vi "Host Image Acquisition Loop.vi"(8 "error in":errorcluster, 11 "Image Reference":refnum<vi>) -> (0 "error out":errorcluster)   [LabVIEW 2013]
doc: "Loop handles the matlab tcp communications.\nInitialize - Queues up the intialize states\nWait For Connection - Calls the TCP module and waits for a connection to be established\nRead Data - Calls the TCP module and reads the data at the port and then parses the command\nCheck Messages - Checks message queue for external messages sent from other threads\nClose Connection - Closes the TCP connection\nExit"
uses:
  Common/State Machines/State Machine Lib.lvlib
  Message Passing/Main MsgQ.lvlib
  Host Image Acquisition Module Enum.ctl
  Message Passing/MsgQ Loops enum.ctl
panel:
  out "FPGA Image":T1(plugin-control)
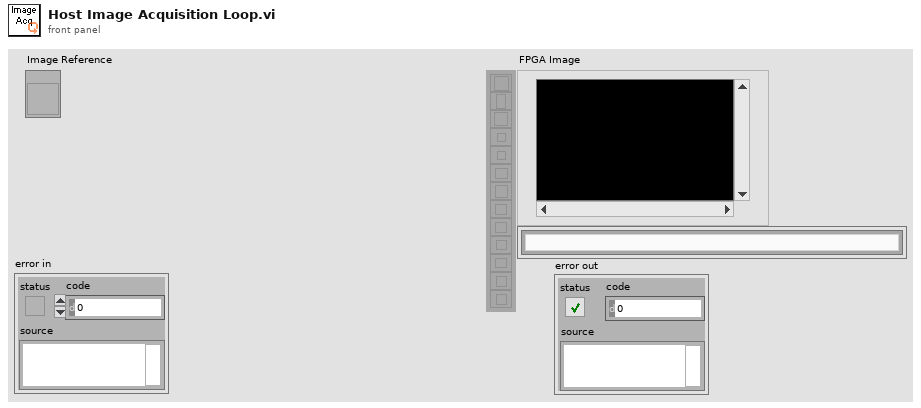
[diagram p1: front panel]
types:
  T1 = typedef "IMAQ Image.ctl" = refnum<image>
  T2 = typedef "State Machine Lib.lvlib/STATE cluster.ctl" = cluster{"State":string, "Parameters":variant}
  T3 = typedef "Host Image Acquisition Module Enum.ctl" = enum16{"Open FPGA", "Initialize DMA FIFO", "Start Acquisition", "Aquire Image", "Close FPGA"}
  T4 = typedef "Main MsgQ.lvlib/MsgQ Loops enum.ctl" = enum16{"User Interface", "Image Acq"}
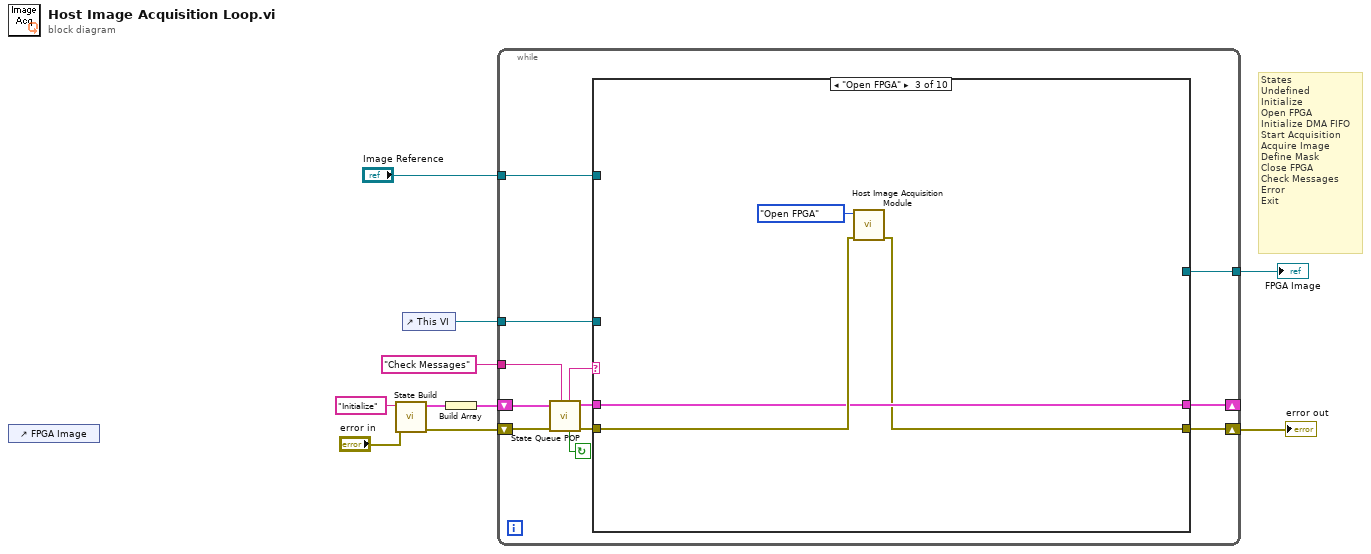
[diagram p0: block diagram]
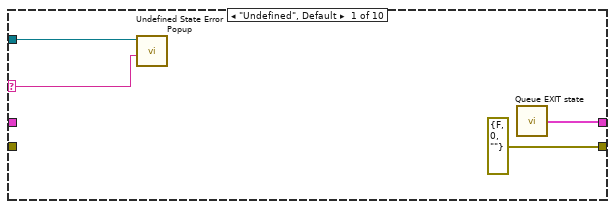
[diagram p2: hidden frame]
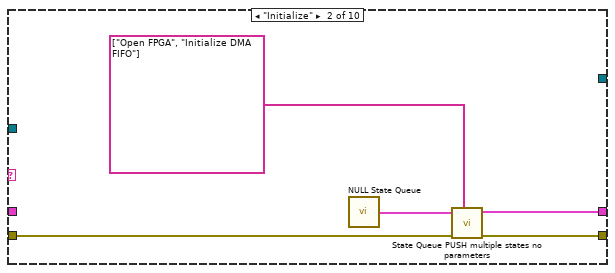
[diagram p3: hidden frame]
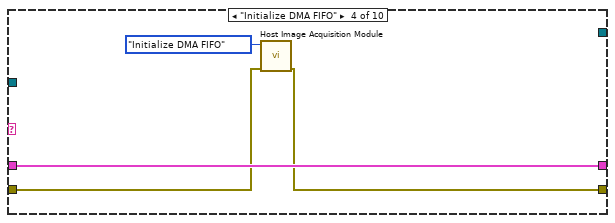
[diagram p4: hidden frame]
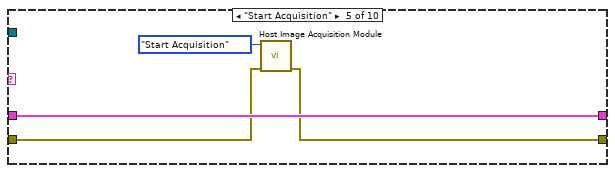
[diagram p5: hidden frame]
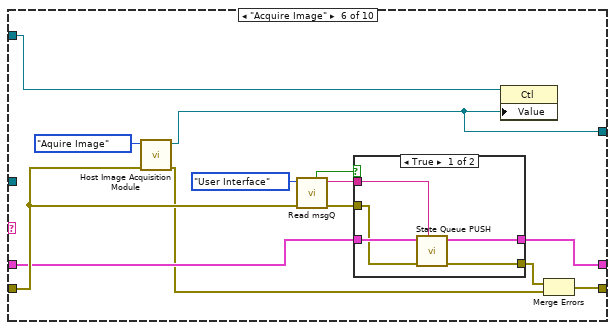
[diagram p6: hidden frame]
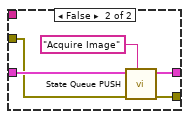
[diagram p7: hidden frame]
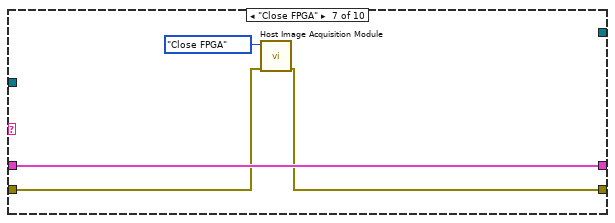
[diagram p8: hidden frame]
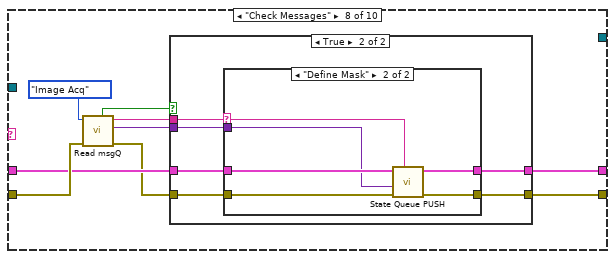
[diagram p9: hidden frame]
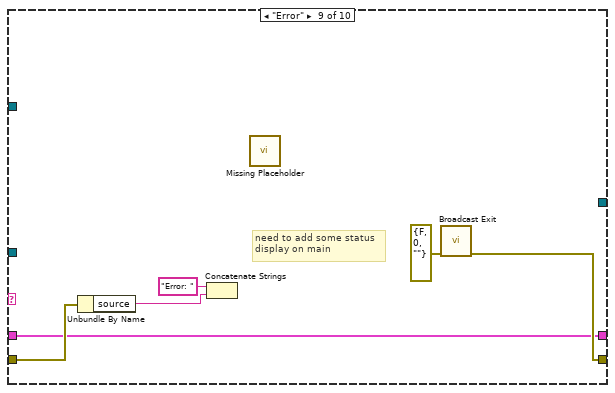
[diagram p12: hidden frame]
diagram:
  # "States\nUndefined\nInitialize\nOpen FPGA\nInitialize DMA FIFO\nStart Acquisition\nAcquire Image\nDefine Mask\nClose FPGA\nCheck Messages\nError\nExit"
  n1 = control-ref of="FPGA Image"() -> ()  [unwired: 1 out]
  n2 = call "State Build.vi"("error in (no error)"="error in", "State"="Initialize") -> ("error out"=w6:errorcluster, "State Out"=w8:T2)  [unwired: 8 in]
  n3 = control-ref of="This VI"() -> (w3:refnum<vi>)
  n4 = Build Array(w8) -> (w7:T2[])
  n5 = while {
    shift-right: [w15] -> _
    shift-left: w7 -> [w22]
    shift-right: [w14] -> w4
    shift-left: w6 -> [w21]
    tunnel: "Check Messages" ("Default state") -> [w19]
    tunnel: w3 -> [w13]
    tunnel: "Image Reference" -> [w12]
    tunnel: [w11] -> w1
    stop <- w20 continue-if-true
    n6 = call "State Queue POP.vi"("Default state"=w19, "error in (no error)"=w21, "State que in"=w22) -> ("error out"=w16:errorcluster, "State que out"=w17:T2[], "Not Exit?"=w20:bool, "State case out"=w18:string)  [unwired: 4 in, 1 out]
    n7 = case shown="\"Open FPGA\"" w18 {
      selector: w18 -> [w25 _ _ _ _ _ _ _ _ _]
      tunnel: w17 -> [_ _ w33 w39 w43 w50 w70 w77 w94 w101]
      tunnel: w16 -> [_ w31 w34 w38 w42 w53 w69 w79 w97 w100]
      tunnel: [w24 w28 w33 w39 w43 w49 w70 w76 w94 w101] -> w15
      tunnel: [errorcluster {"status"=FALSE, "code"=0, "source"=""} ("error out") w27 w32 w37 w41 w46 w68 w75 w95 w100] -> w14
      tunnel: w13 -> [w26 _ _ _ _ _ _ _ _ _]
      tunnel: w12 -> [_ _ _ _ _ w45 _ _ _ _]
      tunnel: [_ _ _ _ _ w44 _ _ _ _] -> w11
      frame "Undefined", Default {
        n8 = call "Undefined State Error Popup.vi"("String"=w25, "This VI (Caller if unwired)"=w26) -> ()  [unwired: 10 in]
        n9 = call "Queue EXIT state.vi"() -> ("Exit State Q"=w24:T2[])  [unwired: 1 in]
      }
      frame "Initialize" {
        n10 = call "NULL State Queue.vi"() -> ("NULL State Queue"=w30:T2[])
        n11 = call "State Queue PUSH multiple states no parameters.vi"("States to queue"=string[] ["Open FPGA", "Initialize DMA FIFO"], "error in (no error)"=w31, "State que in"=w30) -> ("error out"=w27:errorcluster, "State que out"=w28:T2[])  [unwired: 7 in]
      }
      frame "Open FPGA" {
        n12 = call "Host Image Acquisition Module.vi"("error in"=w34, "Operation"=Host_Image_Acquisition_Module_Enum."Open FPGA") -> ("error out"=w32:errorcluster)  [unwired: 8 in, 1 out]
      }
      frame "Initialize DMA FIFO" {
        n13 = call "Host Image Acquisition Module.vi"("error in"=w38, "Operation"=Host_Image_Acquisition_Module_Enum."Initialize DMA FIFO") -> ("error out"=w37:errorcluster)  [unwired: 8 in, 1 out]
      }
      frame "Start Acquisition" {
        n14 = call "Host Image Acquisition Module.vi"("error in"=w42, "Operation"=Host_Image_Acquisition_Module_Enum."Start Acquisition") -> ("error out"=w41:errorcluster)  [unwired: 8 in, 1 out]
      }
      frame "Acquire Image" {
        n15 = call "Host Image Acquisition Module.vi"("error in"=w53, "Operation"=Host_Image_Acquisition_Module_Enum."Aquire Image") -> ("error out"=w47:errorcluster, "Image"=w44:T1)  [unwired: 8 in]
        n16 = call "Read msgQ.vi"("error in"=w53, "MsgQ enum"=MsgQ_Loops_enum."User Interface") -> ("error out"=w51:errorcluster, "Message Received String"=w52:string, "Message Recieved?"=w54:bool)  [unwired: 6 in, 1 out]
        n17 = case shown="True" w54 {
          tunnel: w52 -> [w60 _]
          tunnel: w51 -> [w59 w65]
          tunnel: w50 -> [w61 w66]
          tunnel: [w58 w64] -> w48
          tunnel: [w57 w63] -> w49
          frame True {
            n18 = call "State Queue PUSH.vi"("State case"=w60, "error in (no error)"=w59, "State que in"=w61) -> ("error out"=w58:errorcluster, "State que out"=w57:T2[])  [unwired: 7 in]
          }
          frame False {
            n19 = call "State Queue PUSH.vi"("State case"="Acquire Image", "error in (no error)"=w65, "State que in"=w66) -> ("error out"=w64:errorcluster, "State que out"=w63:T2[])  [unwired: 7 in]
          }
        }
        n20 = property class="Ctl"(reference=w45, "Value"=w44) -> ()  [unwired: 1 in, 2 out]
        n21 = Merge Errors(w48, w47) -> (w46:errorcluster)
      }
      frame "Close FPGA" {
        n22 = call "Host Image Acquisition Module.vi"("error in"=w69, "Operation"=Host_Image_Acquisition_Module_Enum."Close FPGA") -> ("error out"=w68:errorcluster)  [unwired: 8 in, 1 out]
      }
      frame "Check Messages" {
        n23 = call "Read msgQ.vi"("error in"=w79, "MsgQ enum"=MsgQ_Loops_enum."Image Acq") -> ("error out"=w74:errorcluster, "Message Received Parameters"=w71:variant, "Message Received String"=w73:string, "Message Recieved?"=w78:bool)  [unwired: 6 in]
        n24 = case shown="True" w78 {
          tunnel: w77 -> [w81 w87]
          tunnel: [w81 w86] -> w76
          tunnel: [w80 w85] -> w75
          tunnel: w74 -> [w80 w84]
          tunnel: w73 -> [_ w82]
          tunnel: w71 -> [_ w83]
          frame False {
          }
          frame True {
            n25 = case shown="\"Define Mask\"" w82 {
              selector: w82 -> [_ w88]
              tunnel: w87 -> [_ w93]
              tunnel: [_ w92] -> w86
              tunnel: [_ w91] -> w85
              tunnel: w84 -> [_ w90]
              tunnel: w83 -> [_ w89]
              frame "False", Default {
              }
              frame "Define Mask" {
                n26 = call "State Queue PUSH.vi"("State case"=w88, "error in (no error)"=w90, "Parameters"=w89, "State que in"=w93) -> ("error out"=w91:errorcluster, "State que out"=w92:T2[])  [unwired: 6 in]
              }
            }
          }
        }
      }
      frame "Error" {
        # "need to add some status\ndisplay on main"
        n27 = Unbundle By Name(w97) -> ("source"=w98:string)
        n28 = Concatenate Strings("Error: " ("string"), w98) -> ()  [unwired: 1 out]
        n29 = call "Missing Placeholder.vi"() -> ()  [unwired: 12 in]
        n30 = call "Broadcast Exit.vi"("error in"=errorcluster {"status"=FALSE, "code"=0, "source"=""}) -> ("error out"=w95:errorcluster)  [unwired: 10 in]
      }
      frame "Exit" {
      }
    }
  }
  "error out" <- w4
  "FPGA Image" <- w1
